vi "edge_count.vi"(4 "Ultimo RPM encoder":dbl, 6 "RPM setpoint":dbl, 8 "malha controle?":bool, 9 "RPM Samples (n)":i32=25000, 10 "1/rate":dbl, 11 "Data":dbl[](array[numeric])) -> (2 "RPM encoder":dbl, 3 "RPM":dbl)   [LabVIEW 2019]
uses:
  <vilib>/Analysis/baseanly.llb/Mean (DBL).vi
  <vilib>/Analysis/NI_AALBase.lvlib
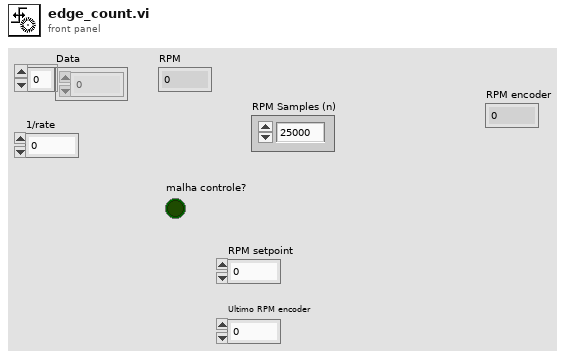
[diagram p1: front panel]
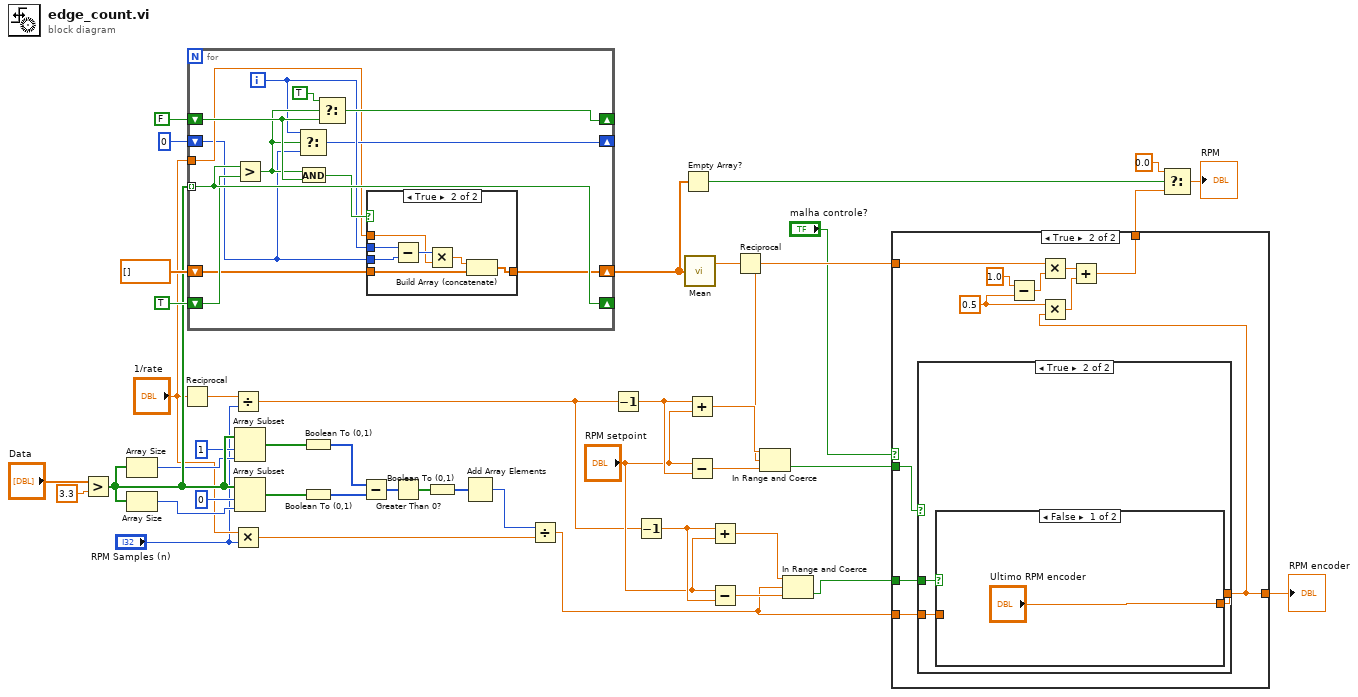
[diagram p0: block diagram]
diagram:
  n1 = Greater?(x="Data", y=3.3) -> (0:w32:bool[])
  n2 = Array Size(array=w32) -> (size(s)=w29:i32)
  n3 = Array Size(array=w32) -> (size(s)=w28:i32)
  n4 = Reciprocal(x="1/rate") -> (1/x=w15:dbl)
  n5 = for {
    tunnel: w32 -> [w56] mode=indexing
    shift-right: [w56] -> _
    shift-left: TRUE -> [w55]
    shift-right: [w51] -> _
    shift-left: FALSE -> [w52]
    shift-right: [w48] -> _
    shift-left: 0 -> [w46]
    tunnel: "1/rate" -> [w47]
    shift-right: [w45] -> w42
    shift-left: dbl[] [] -> [w44]
    i -> [w49]
    n6 = Greater?(x=w56, y=w55) -> (0:w50:bool)
    n7 = Select(t=w49, s=w50, f=w46) -> (s? t:f=w48:i32)
    n8 = And(x=w50, y=w52) -> (x .and. y?=w53:bool)
    n9 = Select(t=TRUE, s=w50, f=w52) -> (s? t:f=w51:bool)
    n10 = case shown="True" w53 {
      tunnel: w49 -> [_ w64]
      tunnel: w46 -> [_ w63]
      tunnel: w47 -> [_ w61]
      tunnel: [w57 w59] -> w45
      tunnel: w44 -> [w57 w58]
      frame False {
      }
      frame True {
        n11 = Subtract(x=w64, y=w63) -> (x-y=w62:i32)
        n12 = Multiply(x=w62, y=w61) -> (x*y=w60:dbl)
        n13 = Build Array (concatenate)(w60, w58) -> (w59:dbl[])
      }
    }
  }
  n14 = Divide(x=w15, y="RPM Samples (n)") -> (x/y=w1:dbl)
  n15 = Multiply(x="1/rate", y="RPM Samples (n)") -> (x*y=w18:dbl)
  n16 = Array Subset(array=w32, index=1, length=w29) -> (w26:bool[])
  n17 = Array Subset(array=w32, index=0, length=w28) -> (w25:bool[])
  n18 = Boolean To (0,1)(Boolean=w26) -> (0, 1=w24:i16[])
  n19 = Boolean To (0,1)(Boolean=w25) -> (0, 1=w23:i16[])
  n20 = Subtract(x=w24, y=w23) -> (x-y=w22:i16[])
  n21 = Greater Than 0?(x=w22) -> (x > 0?=w21:bool[])
  n22 = Boolean To (0,1)(Boolean=w21) -> (0, 1=w20:i16[])
  n23 = Add Array Elements(numeric array=w20) -> (sum=w19:i16)
  n24 = Divide(x=w19, y=w18) -> (x/y=w6:dbl)
  n25 = Decrement(x=w1) -> (x-1=w14:dbl)
  n26 = Decrement(x=w1) -> (x-1=w8:dbl)
  n27 = Empty Array?(array=w42) -> (empty?=w41:bool)
  n28 = call-poly <vilib>:"Mean.vi"("X"=w42) -> ("mean"=w39:dbl)  [unwired: 1 out]
  n29 = Add(x=w14, y="RPM setpoint") -> (x+y=w13:dbl)
  n30 = Subtract(x="RPM setpoint", y=w14) -> (x-y=w12:dbl)
  n31 = Add(x=w8, y="RPM setpoint") -> (x+y=w9:dbl)
  n32 = Subtract(x="RPM setpoint", y=w8) -> (x-y=w10:dbl)
  n33 = Reciprocal(x=w39) -> (1/x=w11:dbl)
  n34 = In Range and Coerce(upper limit=w13, x=w11, lower limit=w12) -> (In Range?=w2:bool)  [unwired: 1 out]
  n35 = In Range and Coerce(upper limit=w9, x=w6, lower limit=w10) -> (In Range?=w4:bool)  [unwired: 1 out]
  n36 = case shown="True" "malha controle?" {
    tunnel: [w65 w77] -> w31
    tunnel: w11 -> [w65 w71]
    tunnel: w6 -> [w66 w69]
    tunnel: [w66 w67] -> w5
    tunnel: w4 -> [_ w70]
    tunnel: w2 -> [_ w68]
    frame False {
    }
    frame True {
      w74 = 0.5
      n37 = case shown="True" w68 {
        tunnel: w70 -> [_ w81]
        tunnel: [w78 w80] -> w67
        tunnel: w69 -> [w78 w79]
        frame False {
        }
        frame True {
          n38 = case shown="False" w81 {
            tunnel: ["Ultimo RPM encoder" w83] -> w80
            tunnel: w79 -> [_ w83]
            frame False {
            }
            frame True {
            }
          }
        }
      }
      n39 = Subtract(x=1.0, y=w74) -> (x-y=w72:dbl)
      n40 = Multiply(x=w71, y=w72) -> (x*y=w76:dbl)
      n41 = Multiply(x=w74, y=w67) -> (x*y=w75:dbl)
      n42 = Add(x=w76, y=w75) -> (x+y=w77:dbl)
    }
  }
  "RPM encoder" <- w5
  n43 = Select(t=0.0, s=w41, f=w31) -> (s? t:f=→"RPM":dbl)
